vi "GenerateTargetPos.vi"(0 "Piece":i32, 1 "Clust Refnum":refnum<vi>, 5 "Index":i32, 7 "Board":i32[][](array[numeric])=[[-3, -5, -4, -2, -1, -4, -5, -3], [-6, -6, -6, -6, -6, -6, -6, -6], [0, 0, 0, 0, 0, 0, 0, 0], [0, 0, 0, 0, 0, 0, 0, 0], [0, 0, 0, 0, 0, 0, 0, 0], [0, 0, 0, 0, 0, 0, 0, 0], [6, 6, 6, 6, 6, 6, 6, 6], [3, 5, 4, 2, 1, 4, 5, 3]], 9 "Black/White Turn (T/F)":bool, 11 "Castling State":bool[][](array[boolean]), 12 "LastMovePiece":cluster{"Row":i32, "Column":i32, "IsMove":bool}) -> (6 "AttachablePosition":bool[][](array[boolean]), 10 "AttachablePositionIndexes":i32[](array[numeric]))   [LabVIEW 2014]
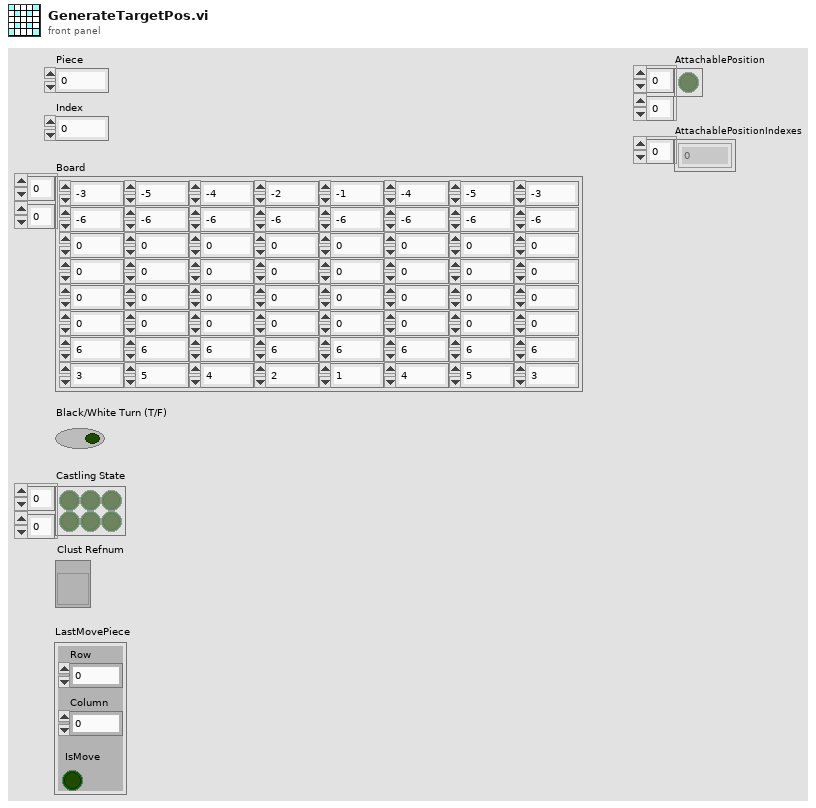
[diagram p1: front panel]
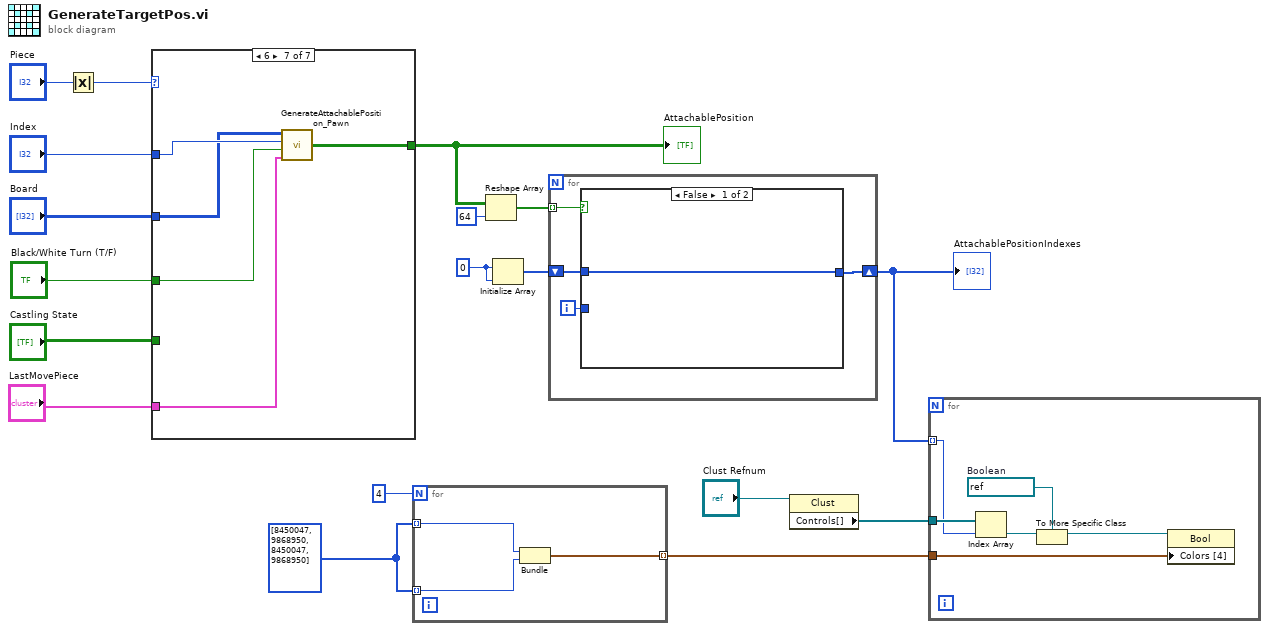
[diagram p0: block diagram]
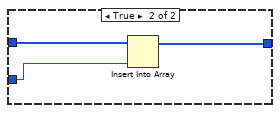
[diagram p2: hidden frame]
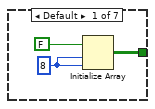
[diagram p3: hidden frame]
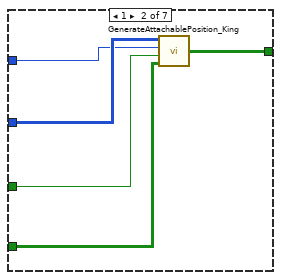
[diagram p4: hidden frame]
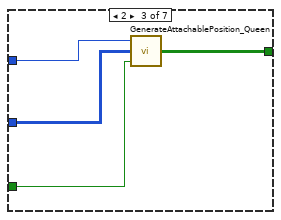
[diagram p5: hidden frame]
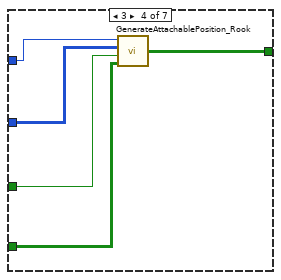
[diagram p6: hidden frame]
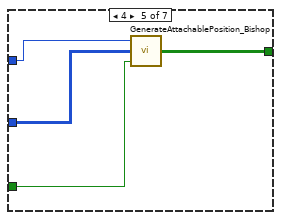
[diagram p7: hidden frame]
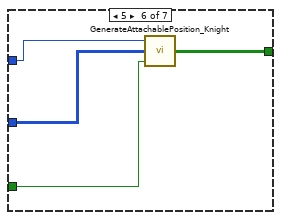
[diagram p8: hidden frame]
diagram:
  w4 = u32[] [8450047, 9868950, 8450047, 9868950] ("Array 3")
  w9 = 0 ("element")
  n1 = Absolute Value(x="Piece") -> (abs(x)=w17:i32)
  n2 = case shown="6" w17 {
    tunnel: "Index" -> [_ w25 w29 w32 w36 w40 w46]
    tunnel: "Board" -> [_ w26 w28 w33 w37 w41 w45]
    tunnel: "Black/White Turn (T/F)" -> [_ w24 w27 w34 w38 w42 w47]
    tunnel: "Castling State" -> [_ w23 _ w31 _ _ _]
    tunnel: [w19 w22 w30 w35 w39 w43 w48] -> w12
    tunnel: "LastMovePiece" -> [_ _ _ _ _ _ w44]
    frame Default {
      w20 = 8
      n3 = Initialize Array(FALSE, w20, w20) -> (w19:bool[][])
    }
    frame 1 {
      n4 = call "GenerateAttachablePosition_King.vi"("Castling State"=w23, "Black/White Turn (T/F)"=w24, "pieceIndex"=w25, "Board"=w26) -> ("AttachablePosition"=w22:bool[][])
    }
    frame 2 {
      n5 = call "GenerateAttachablePosition_Queen.vi"("Black/White Turn (T/F)"=w27, "Board"=w28, "pieceIndex"=w29) -> ("AttachablePosition"=w30:bool[][])
    }
    frame 3 {
      n6 = call "GenerateAttachablePosition_Rook.vi"("Castling State"=w31, "Black/White Turn (T/F)"=w34, "Board"=w33, "pieceIndex"=w32) -> ("AttachablePosition"=w35:bool[][])
    }
    frame 4 {
      n7 = call "GenerateAttachablePosition_Bishop.vi"("Black/White Turn (T/F)"=w38, "Board"=w37, "pieceIndex"=w36) -> ("AttachablePosition"=w39:bool[][])
    }
    frame 5 {
      n8 = call "GenerateAttachablePosition_Knight.vi"("Black/White Turn (T/F)"=w42, "Board"=w41, "pieceIndex"=w40) -> ("AttachablePosition"=w43:bool[][])
    }
    frame 6 {
      n9 = call "GenerateAttachablePosition_Pawn.vi"("LastMovePiece"=w44, "Black/White (T/F)"=w47, "pieceIndex"=w46, "Board"=w45) -> ("AttachablePosition"=w48:bool[][])
    }
  }
  "AttachablePosition" <- w12
  n10 = for {
    N: 4 -> [_]
    tunnel: w4 -> [w50] mode=indexing
    tunnel: w4 -> [w49] mode=indexing
    tunnel: [w51] -> w3 mode=indexing
    n11 = Bundle("Color Box"=w50, "Color Box"=w49) -> (w51:cluster{"Color Box":u32, "Color Box":u32})  [unwired: 1 in]
  }
  n12 = Reshape Array(w12, 64 ("dimension size")) -> (w10:bool[])
  n13 = Initialize Array(w9, w9) -> (w8:i32[])
  n14 = for {
    tunnel: w10 -> [w55] mode=indexing
    shift-right: [w52] -> w7
    shift-left: w8 -> [w53]
    i -> [w54]
    n15 = case shown="False" w55 {
      tunnel: w54 -> [_ w59]
      tunnel: w53 -> [w56 w58]
      tunnel: [w56 w57] -> w52
      frame False {
      }
      frame True {
        n16 = Insert Into Array(array=w58, new element=w59) -> (w57:i32[])  [unwired: 1 in]
      }
    }
  }
  "AttachablePositionIndexes" <- w7
  n17 = property class="Clust"(reference="Clust Refnum") -> ("Controls[]"=w1:refnum<vi>[])  [unwired: 1 in, 2 out]
  n18 = for {
    tunnel: w7 -> [w64] mode=indexing
    tunnel: w1 -> [w65]
    tunnel: w3 -> [w60]
    w62 = refnum<vi> refnum  # Boolean
    n19 = Index Array(array=w65, index=w64) -> (element=w63:refnum<vi>)
    n20 = To More Specific Class(target class=w62, reference=w63) -> (specific class reference=w61:refnum<vi>)  [unwired: 1 in, 1 out]
    n21 = property class="Bool"(reference=w61, "Colors [4]"=w60) -> ()  [unwired: 1 in, 2 out]
  }
